vi "NewJoyPrepare.vi"(11 "Joystick Values":T1) -> (0 "Buttons":T2, 1 "Z Axis":dbl, 2 "Right Stick":dbl, 3 "Left Stick":dbl)   [LabVIEW 2016]
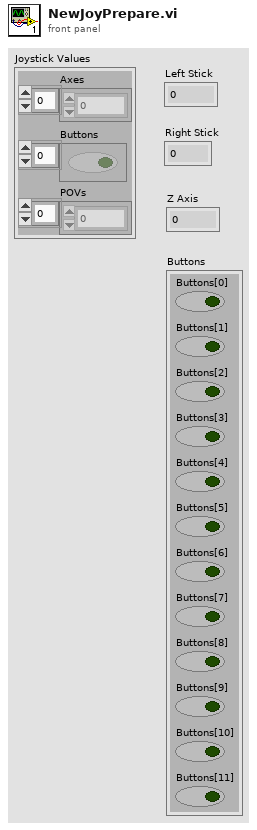
[diagram p1: front panel]
types:
  T1 = cluster{"Axes":dbl[], "Buttons":bool[], "POVs":i16[]}
  T2 = cluster{"Buttons[0]":bool, "Buttons[1]":bool, "Buttons[2]":bool, "Buttons[3]":bool, "Buttons[4]":bool, "Buttons[5]":bool, "Buttons[6]":bool, "Buttons[7]":bool, "Buttons[8]":bool, "Buttons[9]":bool, "Buttons[10]":bool, "Buttons[11]":bool}
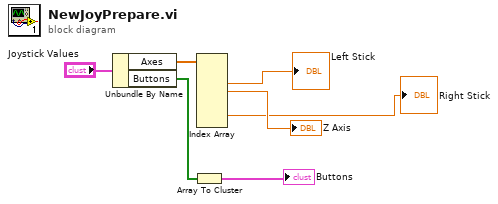
[diagram p0: block diagram]
diagram:
  n1 = Unbundle By Name("Joystick Values") -> ("Axes"=w4:dbl[], "Buttons"=w6:bool[])
  n2 = Array To Cluster(array=w6) -> (cluster=→"Buttons":T2)
  n3 = Index Array(array=w4) -> (element #2=→"Left Stick":dbl, element #3=→"Z Axis":dbl, element #6=→"Right Stick":dbl)  [unwired: 7 in, 4 out]
